vi "Run.vi"(2 "DebugOut":refnum<k21>, 8 "error in (no error)":errorcluster, 10 "Command FIFO":refnum<k21>, 11 "MPU in":refnum<class "MPU.lvclass">) -> (0 "error out":errorcluster, 3 "MPU out":refnum<class "MPU.lvclass">)   [LabVIEW 2018, in "Modbus_Processing_Unit.lvlib" / "MPU.lvclass"]
uses:
  MPU.lvclass
  MPU.lvclass/MPU.ctl
  <vilib>/rvi/Emulation/niFpgaGetClockAttributes.vi
  <vilib>/rvi/Emulation/niFpgaSctlEmulationGetInTimedLoop.vi
  <vilib>/rvi/Emulation/niFpgaEmulationReportErrorSimple.vi
  <vilib>/rvi/DataTransferAndStorage/Container/Common/niFpgaContainerExecOnDevCompGetState.vi
  <vilib>/rvi/Emulation/niFpgaEmulationIsFPGAContextNoSignature.vi
  <vilib>/rvi/errors/niFpgaSetErrorForExecOnDevCompSimple.vi
  <vilib>/rvi/eio/common/nirviEmuReportErrorAndStop.vi
  <vilib>/rvi/DataTransferAndStorage/Container/Common/niFpgaContainerGetUniqueNameForEmu.vi
  <vilib>/rvi/FIFO/Fifo_Resource/nirvififoEmulationSetSize.vi
  <vilib>/rvi/FIFO/Fifo_Resource/nirviFifoEmulationQueueMgr.vi
  <instcachedir>/0/nirviFifoEmulationQueueMgr_E5CAEC123FF24DC58D834DCA3CDAA9B5.lvgen/nirviFifoEmulationQueueMgr_E5CAEC123FF24DC58D834DCA3CDAA9B5_001.vi
  <vilib>/rvi/FIFO/Fifo_Resource/nirvififoEmulationDetermineInputValidOut.vi
  <vilib>/rvi/FIFO/Fifo_Resource/nirvififoEmulationCreateLock.vi
  <vilib>/rvi/Emulation/niFpgaProcessEmulError.vi
  <vilib>/rvi/FIFO/Fifo_Resource/nirvififoEmulationObtainLock.vi
  <vilib>/rvi/FIFO/Fifo_Resource/nirvififoEmulationReleaseLock.vi
  <vilib>/rvi/occurrence/nirviWaitOnOccurrenceBase.vi
  <vilib>/rvi/errors/nirviReportUnexpectedCaseInternalError.vi
  <vilib>/rvi/errors/nirviReportUnexpectedCaseInternalError (U32).vi
  <vilib>/Utility/error.llb/Clear Errors.vi
  <vilib>/rvi/interface/RandomDataEmulation/niFpgaRandomDataHandleErrors.vi
  <vilib>/rvi/Emulation/niFpgaCriticalErrorInLSC.vi
  <vilib>/rvi/DataTransferAndStorage/Container/XNode/niFpgaContainer.xnode
  <vilib>/rvi/FIFO/Fifo_Resource/niFpgaFifoEmulationRefIn.vi
panel:
  # "This is the main method of the class. If new commands (length + commands) are available on CommandFIFO, those becomes the new commands stored in an internal Instructions array. Otherwise, execute the commands. Write Port and Read Port VIs are used to write and read to serial port - those can be overloaded\nas needed. Set Port VI sets the ports for default Write Port and Read Port methods."
  # "Commands:\n0 - stop executing until new commands are loaded\n1 - write the next byte to port\n2 - wait for given ms\n3 - read from port\n4- restart processing\n5 - check data CRC, assumes CRC is last two bytes\n6 - write data to output FIFO\n255 - stop execution, exit the method"
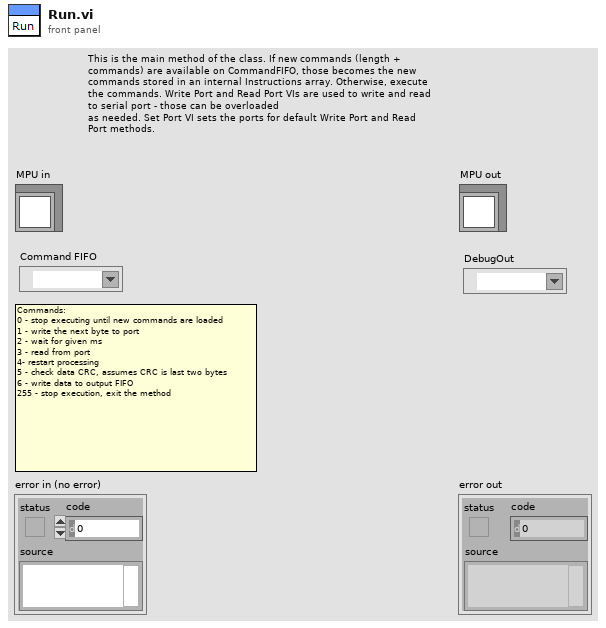
[diagram p1: front panel]
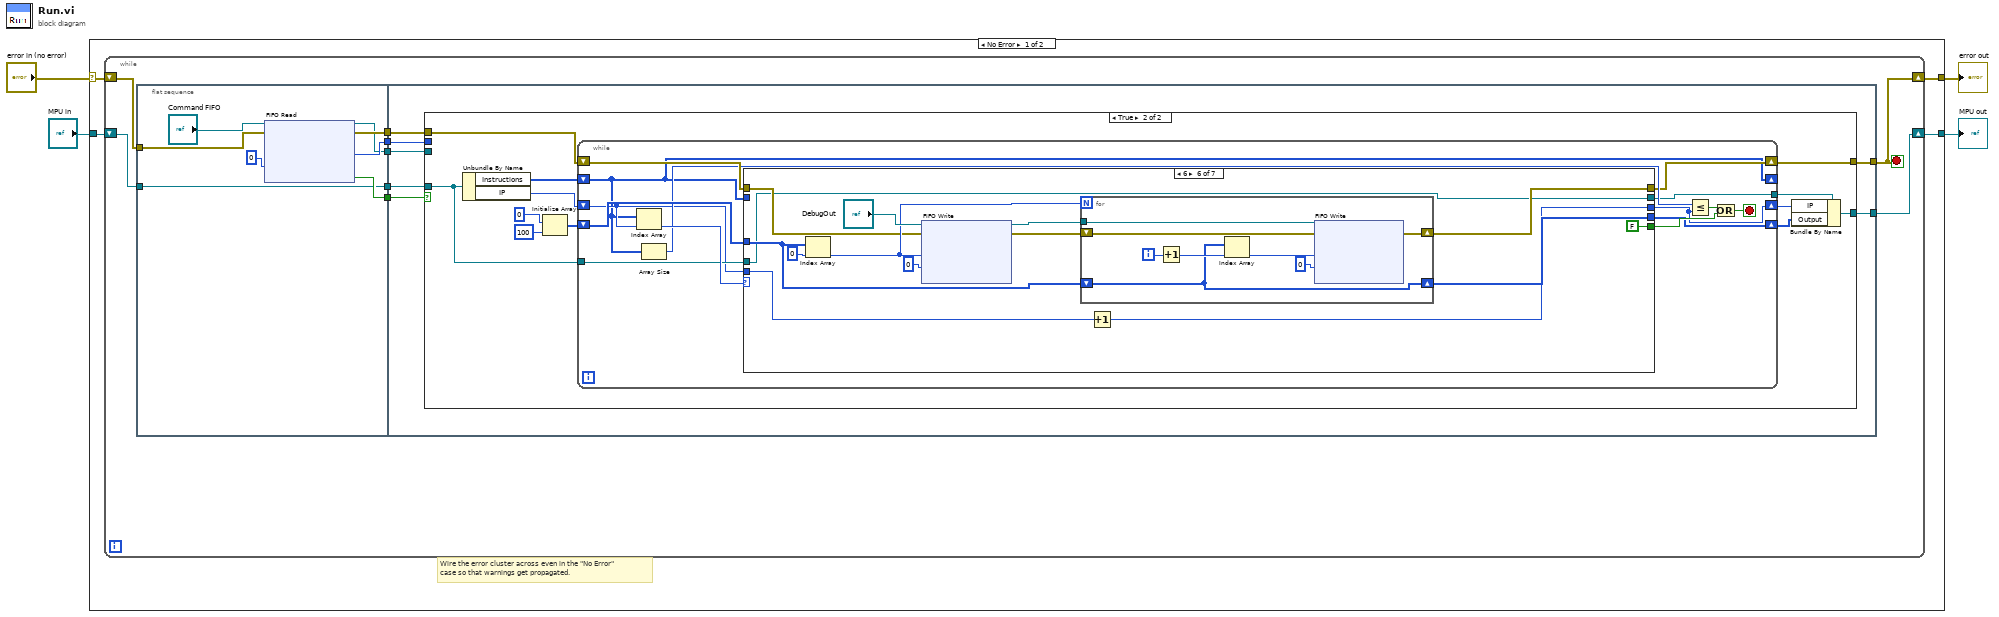
[diagram p0: block diagram]
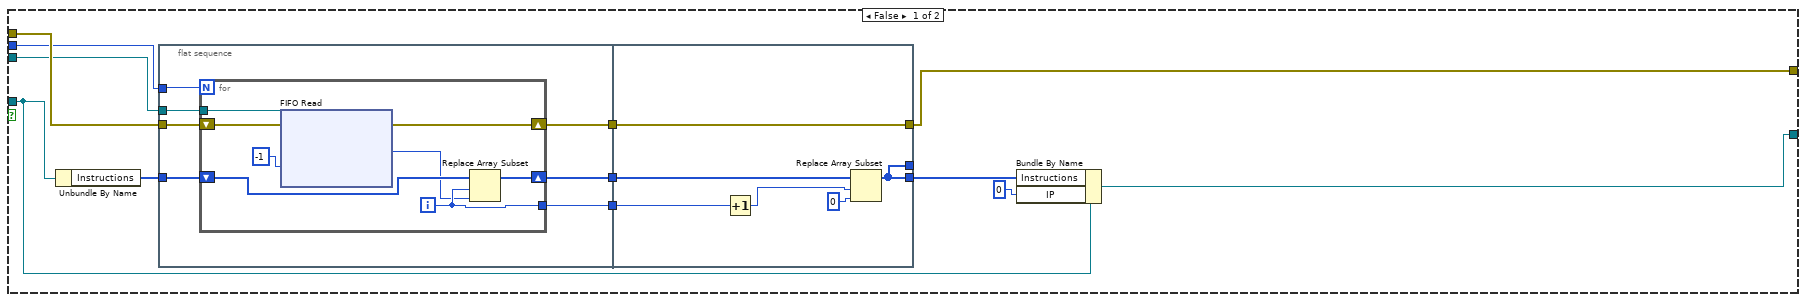
[diagram p2: hidden frame]
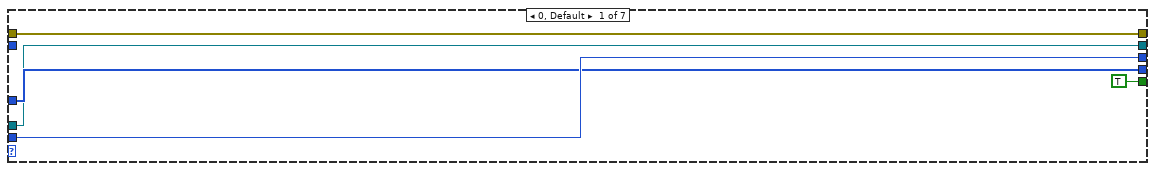
[diagram p3: hidden frame]
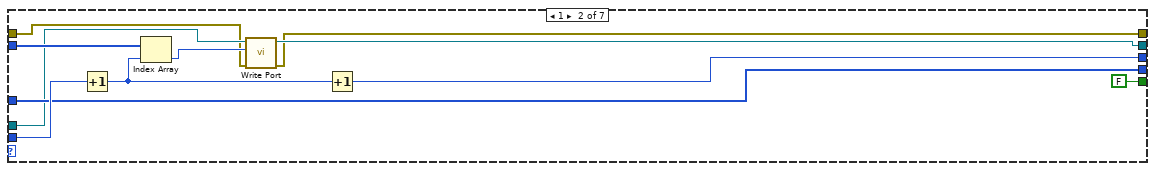
[diagram p4: hidden frame]
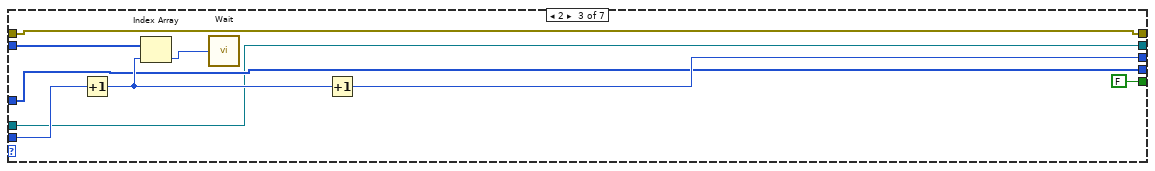
[diagram p5: hidden frame]
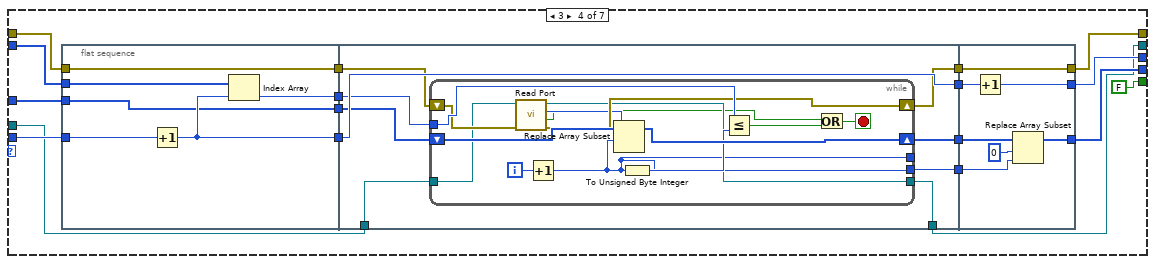
[diagram p6: hidden frame]
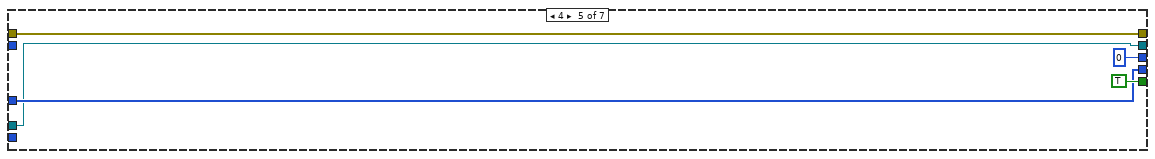
[diagram p7: hidden frame]
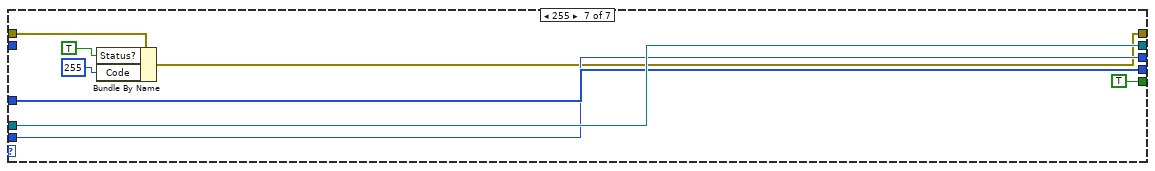
[diagram p8: hidden frame]
diagram:
  n1 = case shown="No Error" "error in (no error)" {
    selector: "error in (no error)" -> [w7 w207]
    tunnel: [w8 w207] -> w4
    tunnel: [w5 w206] -> w3
    tunnel: "MPU in" -> [w6 w206]
    frame No Error {
      # "Wire the error cluster across even in the \"No Error\"\ncase so that warnings get propagated."
      n2 = while {
        shift-right: [w10] -> w8
        shift-left: w7 -> [w17]
        shift-right: [w9] -> w5
        shift-left: w6 -> [w12]
        stop <- w10 stop-if-true
        n3 = flat-sequence {
          tunnel: w17 -> [w25]
          tunnel: [w24] -> w16
          tunnel: [w23] -> w15
          tunnel: [w22] -> w14
          tunnel: [w20] -> w13
          tunnel: w12 -> [w18]
          tunnel: [w18] -> w11
          tunnel: w16 -> [w28]
          tunnel: w15 -> [w32]
          tunnel: w14 -> [w31]
          tunnel: w13 -> [w30]
          tunnel: [w29] -> w10
          tunnel: w11 -> [w27]
          tunnel: [w26] -> w9
          frame #0 {
            n4 = xnode ("FIFO Read")("Timeout"=0, "error in (no error)"=w25, "FIFO In"="Command FIFO") -> ("Element"=w24:u8, "Timed Out?"=w23:bool, "error out"=w22:errorcluster, "FIFO Out"=w20:refnum<k21>)
          }
          frame #1 {
            n5 = case shown="True" w32 {
              tunnel: w31 -> [w44 w77]
              tunnel: w28 -> [w43 _]
              tunnel: w30 -> [w39 _]
              tunnel: [w38 w66] -> w29
              tunnel: w27 -> [w36 w73]
              tunnel: [w35 w70] -> w26
              frame False {
                n6 = Unbundle By Name(w36) -> ("Instructions"=w37:u8[])
                n7 = flat-sequence {
                  tunnel: w43 -> [w49]
                  tunnel: w44 -> [w51]
                  tunnel: [w50] -> w42
                  tunnel: [w45] -> w41
                  tunnel: [w48] -> w40
                  tunnel: w39 -> [w47]
                  tunnel: w37 -> [w46]
                  tunnel: [w65] -> w38
                  tunnel: w42 -> [w65]
                  tunnel: w41 -> [w64]
                  tunnel: w40 -> [w63]
                  tunnel: [w60] -> _
                  tunnel: [w60] -> w34
                  frame #0 {
                    n8 = for {
                      N: w49 -> [_]
                      shift-right: [w58] -> w50
                      shift-left: w51 -> [w59]
                      tunnel: [w55] -> w48
                      tunnel: w47 -> [w54]
                      shift-right: [w52] -> w45
                      shift-left: w46 -> [w57]
                      i -> [w55]
                      n9 = xnode ("FIFO Read")("Timeout"=-1, "error in (no error)"=w59, "FIFO In"=w54) -> ("Element"=w53:u8, "error out"=w58:errorcluster)  [unwired: 2 out]
                      n10 = Replace Array Subset(array=w57, new element=w53, index=w55) -> (w52:u8[])
                    }
                  }
                  frame #1 {
                    n11 = Increment(x=w63) -> (x+1=w62:i32)
                    n12 = Replace Array Subset(array=w64, new element=u8 0 ("new element/subarray"), index=w62) -> (w60:u8[])
                  }
                }
                n13 = Bundle By Name(cluster=w36, "Instructions"=w34, "IP"=i16 0) -> (w35:refnum<class "MPU.lvclass">)
              }
              frame True {
                n14 = Unbundle By Name(w73) -> ("Instructions"=w72:u8[], "IP"=w71:i16)
                n15 = Initialize Array(u8 0 ("element"), 100 ("dimension size")) -> (w74:u8[])
                n16 = while {
                  shift-right: [w87] -> w68
                  shift-left: w74 -> [w88]
                  shift-right: [w81] -> w69
                  shift-left: w71 -> [w82]
                  shift-right: [w79] -> w66
                  shift-left: w77 -> [w90]
                  tunnel: w73 -> [w83]
                  tunnel: [w80] -> w67
                  shift-right: [w78] -> _
                  shift-left: w72 -> [w78]
                  stop <- w86 stop-if-true
                  n17 = Index Array(array=w78, index=w82) -> (element=w89:u8)
                  n18 = Array Size(array=w78) -> (size(s)=w84:i32)
                  n19 = case shown="6" w89 {
                    tunnel: [TRUE FALSE FALSE FALSE TRUE FALSE TRUE] -> w91
                    tunnel: w90 -> [w93 w98 w109 w128 w172 w179 w201]
                    tunnel: w82 -> [w95 w105 w114 w126 _ w184 w203]
                    tunnel: [w95 w103 w113 w133 i16 0 w183 w203] -> w81
                    tunnel: w78 -> [_ w106 w116 w134 _ _ _]
                    tunnel: [w94 w102 w110 w122 w173 w186 w204] -> w87
                    tunnel: w88 -> [w94 w102 w110 w121 w173 w187 w204]
                    tunnel: [w93 w97 w109 w119 w172 w182 w200] -> w79
                    tunnel: w83 -> [w92 w101 w108 w118 w171 w176 w205]
                    tunnel: [w92 w100 w108 w117 w171 w176 w205] -> w80
                    frame 0, Default {
                    }
                    frame 1 {
                      n20 = Increment(x=w105) -> (x+1=w104:i16)
                      n21 = Index Array(array=w106, index=w104) -> (element=w99:u8)
                      n22 = call-dynamic "Write Port.vi"("error in (no error)"=w98, "Data"=w99, "MPU in"=w101) -> ("error out"=w97:errorcluster, "MPU out"=w100:refnum<class "MPU.lvclass">)  [unwired: 6 in, 1 out]
                      n23 = Increment(x=w104) -> (x+1=w103:i16)
                    }
                    frame 2 {
                      n24 = Increment(x=w114) -> (x+1=w112:i16)
                      n25 = Index Array(array=w116, index=w112) -> (element=w115:u8)
                      n26 = call "Wait"("Count(mSec)"=w115) -> ()  [unwired: 1 out]
                      n27 = Increment(x=w112) -> (x+1=w113:i16)
                    }
                    frame 3 {
                      n28 = flat-sequence {
                        tunnel: w134 -> [w140]
                        tunnel: [w139] -> w130
                        tunnel: w128 -> [w138]
                        tunnel: [w138] -> w129
                        tunnel: w126 -> [w137]
                        tunnel: [w136] -> w125
                        tunnel: w121 -> [w135]
                        tunnel: [w135] -> w120
                        tunnel: [w149] -> w132
                        tunnel: [w148] -> w131
                        tunnel: w130 -> [w145]
                        tunnel: w129 -> [w147]
                        tunnel: [w146] -> w127
                        tunnel: w125 -> [w149]
                        tunnel: [w141] -> w123
                        tunnel: w120 -> [w144]
                        tunnel: w118 -> [w143]
                        tunnel: [w142] -> w117
                        tunnel: [w169] -> w119
                        tunnel: [w168] -> w133
                        tunnel: w132 -> [w170]
                        tunnel: w131 -> [w169]
                        tunnel: w127 -> [w167]
                        tunnel: [w166] -> w122
                        tunnel: w123 -> [w165]
                        frame #0 {
                          n29 = Increment(x=w137) -> (x+1=w136:i16)
                          n30 = Index Array(array=w140, index=w136) -> (element=w139:u8)
                        }
                        frame #1 {
                          n31 = while {
                            shift-right: [w155] -> w148
                            shift-left: w147 -> [w156]
                            shift-right: [w163] -> w146
                            shift-left: w144 -> [w162]
                            tunnel: w145 -> [w159]
                            tunnel: w143 -> [w154]
                            tunnel: [w153] -> w142
                            tunnel: [w150] -> _
                            tunnel: [w150] -> w141
                            i -> [w158]
                            stop <- w161 stop-if-true
                            n32 = call-dynamic "Read Port.vi"("error in (no error)"=w156, "MPU in"=w154) -> ("error out"=w155:errorcluster, "Timeouted"=w151:bool, "Data"=w152:u8, "MPU out"=w153:refnum<class "MPU.lvclass">)  [unwired: 6 in]
                            n33 = Increment(x=w158) -> (x+1=w150:i32)
                            n34 = Replace Array Subset(array=w162, new element=w152, index=w150) -> (w163:u8[])
                            n35 = To Unsigned Byte Integer(number=w150) -> (unsigned 8bit integer=w160:u8)
                            n36 = Less Or Equal?(x=w159, y=w160) -> (x <= y?=w157:bool)
                            n37 = Or(x=w151, y=w157) -> (x .or. y?=w161:bool)
                          }
                        }
                        frame #2 {
                          n38 = Increment(x=w170) -> (x+1=w168:i16)
                          n39 = Replace Array Subset(array=w167, new element=w165, index=0) -> (w166:u8[])
                        }
                      }
                    }
                    frame 4 {
                    }
                    frame 6 {
                      n40 = Index Array(array=w187, index=0) -> (element=w180:u8)
                      n41 = xnode "FIFO Write"("Element"=w180, "Timeout"=0, "error in (no error)"=w179, "FIFO In"="DebugOut") -> ("error out"=w178:errorcluster, "FIFO Out"=w181:refnum<k21>)  [unwired: 1 out]
                      n42 = for {
                        N: w180 -> [_]
                        shift-right: [w195] -> w186
                        shift-left: w187 -> [w195]
                        tunnel: w181 -> [w194]
                        shift-right: [w190] -> w182
                        shift-left: w178 -> [w193]
                        i -> [w197]
                        n43 = Increment(x=w197) -> (x+1=w196:i32)
                        n44 = Index Array(array=w195, index=w196) -> (element=w191:u8)
                        n45 = xnode "FIFO Write"("Element"=w191, "Timeout"=0, "error in (no error)"=w193, "FIFO In"=w194) -> ("error out"=w190:errorcluster)  [unwired: 2 out]
                      }
                      n46 = Increment(x=w184) -> (x+1=w183:i16)
                    }
                    frame 255 {
                      n47 = Bundle By Name(cluster=w201, "Status?"=TRUE, "Code"=255) -> (w200:errorcluster)
                    }
                  }
                  n48 = Less Or Equal?(x=w84, y=w81) -> (x <= y?=w85:bool)
                  n49 = Or(x=w85, y=w91) -> (x .or. y?=w86:bool)
                }
                n50 = Bundle By Name(cluster=w67, "IP"=w69, "Output"=w68) -> (w70:refnum<class "MPU.lvclass">)
              }
            }
          }
        }
      }
    }
    frame Error {
    }
  }
  "error out" <- w4
  "MPU out" <- w3
